vi "launch_wait.vi"(8 "error in (no error)":errorcluster, 9 "steps":variant, 10 "recipe_data in":variant, 11 "data":variant) -> (0 "error out":errorcluster)   [LabVIEW 2015, in "example_01.lvlib"]
uses:
  example_01.lvlib
  lv-recipe-machine/public/_controls/transition.ctl
  lv-recipe-machine/public/_controls/error.ctl
  _controls/steps_actions_data.ctl
  _controls/steps_actions.ctl
  lv-recipe-machine/public/_controls/step.ctl
  lv-recipe-machine/public/_controls/vi_reference_type.ctl
  lv-recipe-machine/lv-recipe-machine.lvlib
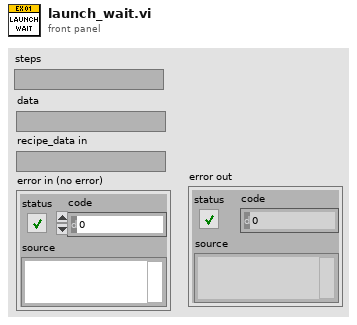
[diagram p1: front panel]
types:
  T1 = typedef "lv-recipe-machine.lvlib/error.ctl" = enum16{"<error>", "bad_command", "command_queue_timeout", "stop_notifier_timeout", "die_command_timeout", "not_in_manual_mode", "not_in_automatic_mode", "not_in_automatic_idle", "not_in_automatic_running", "not_in_automatic_paused", "automatic_step_not_found", "manual_action_not_found", "automatic_not_transition_vi", "transition_step_not_found", "unsupported_vi_type", "<null>"}
  T2 = typedef "lv-recipe-machine.lvlib/step.ctl" = cluster{"name":string, "vi_reference":variant}
  T3 = typedef "example_01.lvlib/steps_actions.ctl" = enum16{"<steps_actions>", "manual_random", "manual_comparison", "manual_wait", "auto_random", "auto_wait", "criteria_initialize", "criteria_count", "criteria_comparison", "transition_simple", "transition_count", "transition_comparison", "launch_wait", "<null>"}
  T4 = typedef "example_01.lvlib/steps_actions_data.ctl" = cluster{"step_action":T3, "data":variant}
  T5 = typedef "lv-recipe-machine.lvlib/transition.ctl" = cluster{"next_index":i32, "data":variant, "recipe_data":variant, "error":errorcluster}
  T6 = typedef "lv-recipe-machine.lvlib/vi_reference_type.ctl" = enum16{"<vi_reference_type>", "manual_action", "auto_step", "auto_criteria", "auto_transition", "auto_launcher", "<null>"}
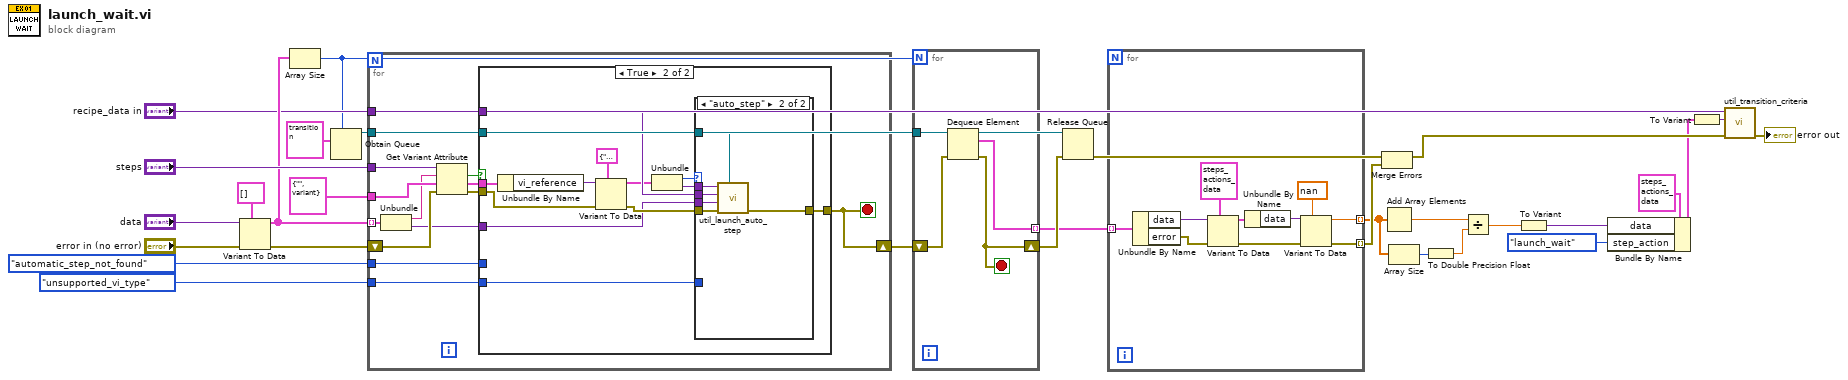
[diagram p0: block diagram]
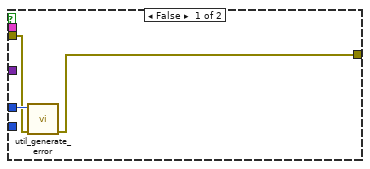
[diagram p2: hidden frame]
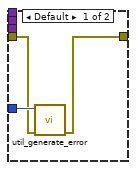
[diagram p3: hidden frame]
diagram:
  n1 = Variant To Data(error in="error in (no error)", type=cluster{"step":string, "data":variant}[] [], Variant="data") -> (data=w23:cluster{"step":string, "data":variant}[], error out=w26:errorcluster)
  n2 = Array Size(array=w23) -> (size(s)=w20:i32)
  n3 = Obtain Queue(max queue size (-1, unlimited)=w20, element data type=T5 {"next_index"=0, "data"=variant, "recipe_data"=variant, "error"={"status"=FALSE, "code"=0, "source"=""}} ("transition")) -> (queue out=w19:refnum<queue>)  [unwired: 3 in, 2 out]
  n4 = for {
    tunnel: w23 -> [w43] mode=indexing
    shift-right: [w32] -> w18
    shift-left: w26 -> [w44]
    tunnel: "steps" -> [w42]
    tunnel: T2 {"name"="", "vi_reference"=variant(refnum<vi> refnum)} ("step") -> [w41]
    tunnel: error."automatic_step_not_found" ("error") -> [w37]
    tunnel: w19 -> [w36]
    tunnel: "recipe_data in" -> [w35]
    tunnel: error."unsupported_vi_type" ("error") -> [w31]
    stop <- w32 stop-if-true
    n5 = Unbundle(w43) -> ("step"=w34:string, "data"=w33:variant)
    n6 = Get Variant Attribute(Variant=w42, name=w34, default value (empty Variant)=w41, error in=w44) -> (found=w40:bool, value=w39:T2, error out=w38:errorcluster)  [unwired: 1 out]
    n7 = case shown="True" w40 {
      tunnel: w39 -> [_ w59]
      tunnel: w38 -> [w46 w53]
      tunnel: w37 -> [w47 _]
      tunnel: w36 -> [_ w58]
      tunnel: w35 -> [_ w57]
      tunnel: w33 -> [_ w56]
      tunnel: [w45 w55] -> w32
      tunnel: w31 -> [_ w48]
      frame False {
        n8 = call "util_generate_error.vi"("error in (no error)"=w46, "error"=w47) -> ("error out"=w45:errorcluster)  [unwired: 9 in]
      }
      frame True {
        n9 = Unbundle By Name(w59) -> ("vi_reference"=w54:variant)
        n10 = Variant To Data(error in=w53, type=cluster{"vi_reference_type":T6, variant} {"vi_reference_type"=enum."<vi_reference_type>", variant}, Variant=w54) -> (data=w51:cluster{"vi_reference_type":T6, variant}, error out=w60:errorcluster)
        n11 = Unbundle(w51) -> ("vi_reference_type"=w49:T6, w50:variant)
        n12 = case shown="\"auto_step\"" w49 {
          tunnel: w58 -> [_ w69]
          tunnel: w57 -> [_ w68]
          tunnel: w56 -> [_ w67]
          tunnel: [w61 w66] -> w55
          tunnel: w50 -> [_ w65]
          tunnel: w48 -> [w63 _]
          tunnel: w60 -> [w62 w64]
          frame Default {
            n13 = call "util_generate_error.vi"("error in (no error)"=w62, "error"=w63) -> ("error out"=w61:errorcluster)  [unwired: 9 in]
          }
          frame "auto_step" {
            n14 = call "util_launch_auto_step.vi"("transition_queue"=w69, "error in (no error)"=w64, "data"=w67, "recipe_data"=w68, "vi_reference"=w65) -> ("error out"=w66:errorcluster)  [unwired: 6 in]
          }
        }
      }
    }
  }
  n15 = for {
    N: w20 -> [_]
    tunnel: w19 -> [w73]
    shift-right: [w71] -> w17
    shift-left: w18 -> [w72]
    tunnel: [w70] -> w16 mode=indexing
    stop <- w71 stop-if-true
    n16 = Dequeue Element(queue=w73, error in (no error)=w72) -> (element=w70:T5, error out=w71:errorcluster)  [unwired: 1 in, 2 out]
  }
  n17 = Release Queue(queue=w19, error in (no error)=w17) -> (error out=w15:errorcluster)  [unwired: 1 in, 2 out]
  n18 = for {
    tunnel: w16 -> [w83] mode=indexing
    tunnel: [w81] -> w3 mode=indexing
    tunnel: [w80] -> w13 mode=indexing
    n19 = Unbundle By Name(w83) -> ("data"=w79:variant, "error"=w78:errorcluster)
    n20 = Variant To Data(error in=w78, type=T4 {"step_action"=enum."<steps_actions>", "data"=variant} ("step_data"), Variant=w79) -> (data=w75:T4, error out=w77:errorcluster)
    n21 = Unbundle By Name(w75) -> ("data"=w74:variant)
    n22 = Variant To Data(error in=w77, type=nan, Variant=w74) -> (data=w81:dbl, error out=w80:errorcluster)
  }
  n23 = Merge Errors(w15, w13) -> (w14:errorcluster)
  n24 = Add Array Elements(numeric array=w3) -> (sum=w11:dbl)
  n25 = Array Size(array=w3) -> (size(s)=w2:i32)
  n26 = To Double Precision Float(number=w2) -> (double precision float=w1:dbl)
  n27 = Divide(x=w11, y=w1) -> (x/y=w4:dbl)
  n28 = To Variant(anything=w4) -> (Variant=w10:variant)
  n29 = Bundle By Name(cluster=T4 {"step_action"=enum."<steps_actions>", "data"=variant}, "data"=w10, "step_action"=steps_actions."launch_wait") -> (w8:T4)
  n30 = To Variant(anything=w8) -> (Variant=w7:variant)
  n31 = call "util_transition_criteria.vi"("error in (no error)"=w14, "data"=w7, "recipe_data"="recipe_data in") -> ("error out"=→"error out":errorcluster)  [unwired: 8 in]
